vi "New Data Point.vi"(8 "error in (no error)":errorcluster, 10 "X":dbl format="%#_13g", 11 "Linear in":refnum<class "Quadratic.lvclass">) -> (0 "error out":errorcluster, 2 "Y(X)":dbl, 3 "Linear out":refnum<class "Quadratic.lvclass">)   [LabVIEW 2020, in "Data Generators.lvlib" / "Quadratic.lvclass"]
uses:
  Quadratic.lvclass
  Quadratic.lvclass/Quadratic.ctl
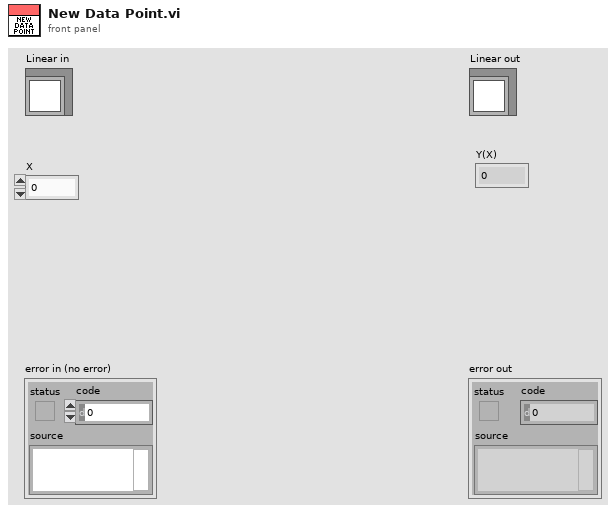
[diagram p1: front panel]
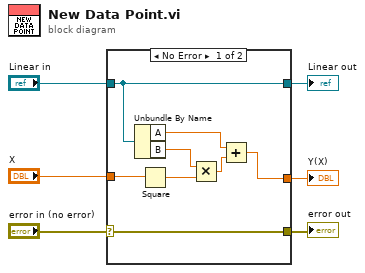
[diagram p0: block diagram]
diagram:
  n1 = case shown="No Error" "error in (no error)" {
    selector: "error in (no error)" -> [w14 w15]
    tunnel: [w14 w15] -> w5
    tunnel: "X" -> [w9 w17]
    tunnel: "Linear in" -> [w13 w16]
    tunnel: [w13 w16] -> w2
    tunnel: [w8 w17] -> w1
    frame No Error {
      n2 = Unbundle By Name(w13) -> ("A"=w12:dbl, "B"=w10:dbl)
      n3 = Square(x=w9) -> (x^2=w7:dbl)
      n4 = Multiply(x=w10, y=w7) -> (x*y=w11:dbl)
      n5 = Add(x=w12, y=w11) -> (x+y=w8:dbl)
    }
    frame Error {
    }
  }
  "error out" <- w5
  "Linear out" <- w2
  "Y(X)" <- w1
